vi "Set Cache Params.vi"(8 "error in (no error)":errorcluster, 10 "Cache Params":T1={"Enabled"=FALSE, "Directive"=enum."None (no-store)", "Max Age"=0, "Immutable"=FALSE, "Last Modified"=timestamp(0 s since 1904-01-01), "Expires"=timestamp(0 s since 1904-01-01), "ETag"="", "Weak ETag"=FALSE}, 11 "Response in":refnum<class "Response.lvclass">) -> (0 "error out":errorcluster, 3 "Response out":refnum<class "Response.lvclass">)   [LabVIEW 2020, in "HTTP Utils.lvlib" / "Response.lvclass"]
uses:
  Response.lvclass
  Cache Params.ctl
  Cache Directive.ctl
  HTTP Utils.lvlib
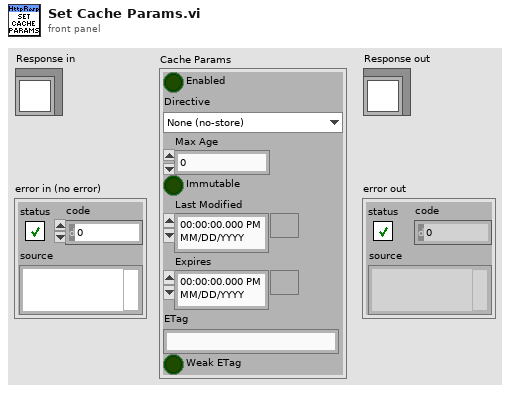
[diagram p1: front panel]
types:
  T1 = typedef "HTTP Utils.lvlib/Cache Params.ctl" = cluster{"Enabled":bool, "Directive":T2, "Max Age":i32, "Immutable":bool, "Last Modified":timestamp, "Expires":timestamp, "ETag":string, "Weak ETag":bool}
  T2 = typedef "HTTP Utils.lvlib/Cache Directive.ctl" = enum16{"Not Specified", "None (no-store)", "Always Validate (no-cache)", "Private Only (private)", "Always Allow (public)"}
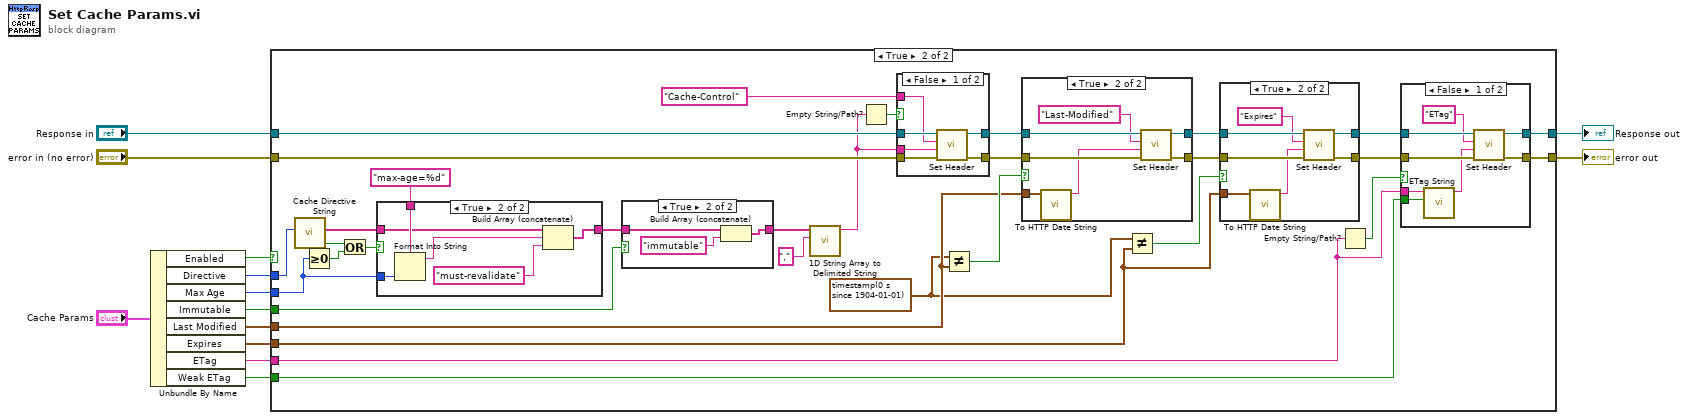
[diagram p0: block diagram]
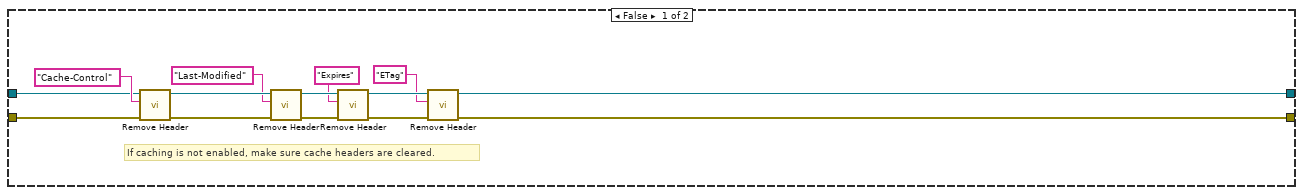
[diagram p2: hidden frame]
diagram:
  n1 = Unbundle By Name("Cache Params") -> ("Enabled"=w12:bool, "Directive"=w11:T2, "Max Age"=w10:i32, "Immutable"=w9:bool, "Last Modified"=w8:timestamp, "Expires"=w7:timestamp, "ETag"=w6:string, "Weak ETag"=w1:bool)
  n2 = case shown="True" w12 {
    tunnel: "error in (no error)" -> [w27 w59]
    tunnel: w11 -> [_ w57]
    tunnel: w10 -> [_ w53]
    tunnel: w9 -> [_ w50]
    tunnel: w8 -> [_ w46]
    tunnel: w7 -> [_ w41]
    tunnel: w6 -> [_ w37]
    tunnel: [w16 w36] -> w5
    tunnel: [w15 w35] -> w4
    tunnel: "Response in" -> [w14 w34]
    tunnel: w1 -> [_ w28]
    frame False {
      # "If caching is not enabled, make sure cache headers are cleared."
      n3 = call "Remove Header.vi"("error in (no error)"=w27, "Header"="Cache-Control", "Response in"=w14) -> ("error out"=w24:errorcluster, "Response out"=w25:refnum<class "Response.lvclass">)  [unwired: 5 in, 2 out]
      n4 = call "Remove Header.vi"("error in (no error)"=w24, "Header"="Last-Modified", "Response in"=w25) -> ("error out"=w21:errorcluster, "Response out"=w22:refnum<class "Response.lvclass">)  [unwired: 5 in, 2 out]
      n5 = call "Remove Header.vi"("error in (no error)"=w21, "Header"="Expires", "Response in"=w22) -> ("error out"=w18:errorcluster, "Response out"=w19:refnum<class "Response.lvclass">)  [unwired: 5 in, 2 out]
      n6 = call "Remove Header.vi"("error in (no error)"=w18, "Header"="ETag", "Response in"=w19) -> ("error out"=w15:errorcluster, "Response out"=w16:refnum<class "Response.lvclass">)  [unwired: 5 in, 2 out]
    }
    frame True {
      w43 = timestamp(0 s since 1904-01-01) ("x")
      n7 = call "Cache Directive String.vi"("Cache Directive"=w57) -> ("Cache-Control Directive"=w56:string[], "no-store?"=w55:bool)  [unwired: 9 in]
      n8 = Greater Or Equal To 0?(x=w53) -> (x >= 0?=w33:bool)
      n9 = Or(x=w55, y=w33) -> (x .or. y?=w54:bool)
      n10 = case shown="True" w54 {
        tunnel: w56 -> [w60 w64]
        tunnel: w53 -> [_ w66]
        tunnel: [w60 w61] -> w51
        tunnel: "max-age=%d" ("string") -> [_ w65]
        frame False {
        }
        frame True {
          n11 = Format Into String(format string=w65, w66) -> (resulting string=w62:string)  [unwired: 2 in, 1 out]
          n12 = Build Array (concatenate)(w64, w62, "must-revalidate" ("string")) -> (w61:string[])
        }
      }
      n13 = case shown="True" w50 {
        tunnel: w51 -> [w103 w106]
        tunnel: [w103 w104] -> w30
        frame False {
        }
        frame True {
          n14 = Build Array (concatenate)(w106, "immutable" ("string")) -> (w104:string[])
        }
      }
      n15 = call <vilib>:"1D String Array to Delimited String.vi"("delimiter"=",", "string array"=w30) -> ("delimited string"=w29:string)  [unwired: 9 in]
      n16 = Empty String/Path?(string/path=w29) -> (empty?=w32:bool)
      n17 = case shown="False" w32 {
        tunnel: w59 -> [w72 w73]
        tunnel: "Cache-Control" ("Header") -> [w67 _]
        tunnel: w29 -> [w71 _]
        tunnel: [w70 w74] -> w48
        tunnel: [w69 w73] -> w47
        tunnel: w34 -> [w68 w74]
        frame False {
          n18 = call "Set Header.vi"("error in (no error)"=w72, "Value"=w71, "Header"=w67, "Response in"=w68) -> ("error out"=w69:errorcluster, "Response out"=w70:refnum<class "Response.lvclass">)  [unwired: 5 in, 1 out]
        }
        frame True {
        }
      }
      n19 = Not Equal?(x=w43, y=w46) -> (x != y?=w49:bool)
      n20 = case shown="True" w49 {
        tunnel: w48 -> [w94 w102]
        tunnel: w47 -> [w95 w101]
        tunnel: w46 -> [_ w99]
        tunnel: [w94 w97] -> w44
        tunnel: [w95 w96] -> w45
        frame False {
        }
        frame True {
          n21 = call "To HTTP Date String.vi"("Time Stamp"=w99) -> ("HTTP Date"=w98:string)  [unwired: 10 in]
          n22 = call "Set Header.vi"("error in (no error)"=w101, "Value"=w98, "Header"="Last-Modified", "Response in"=w102) -> ("error out"=w96:errorcluster, "Response out"=w97:refnum<class "Response.lvclass">)  [unwired: 5 in, 1 out]
        }
      }
      n23 = Not Equal?(x=w43, y=w41) -> (x != y?=w42:bool)
      n24 = case shown="True" w42 {
        tunnel: w45 -> [w85 w91]
        tunnel: w44 -> [w86 w92]
        tunnel: w41 -> [_ w93]
        tunnel: [w86 w88] -> w40
        tunnel: [w85 w87] -> w39
        frame False {
        }
        frame True {
          n25 = call "To HTTP Date String.vi"("Time Stamp"=w93) -> ("HTTP Date"=w90:string)  [unwired: 10 in]
          n26 = call "Set Header.vi"("error in (no error)"=w91, "Value"=w90, "Header"="Expires", "Response in"=w92) -> ("error out"=w87:errorcluster, "Response out"=w88:refnum<class "Response.lvclass">)  [unwired: 5 in, 1 out]
        }
      }
      n27 = Empty String/Path?(string/path=w37) -> (empty?=w38:bool)
      n28 = case shown="False" w38 {
        tunnel: w40 -> [w82 w84]
        tunnel: w39 -> [w81 w83]
        tunnel: w37 -> [w77 _]
        tunnel: [w79 w84] -> w36
        tunnel: [w78 w83] -> w35
        tunnel: w28 -> [w76 _]
        frame False {
          n29 = call "ETag String.vi"("Weak"=w76, "ETag"=w77) -> ("ETag Value"=w75:string)  [unwired: 9 in]
          n30 = call "Set Header.vi"("error in (no error)"=w81, "Value"=w75, "Header"="ETag", "Response in"=w82) -> ("error out"=w78:errorcluster, "Response out"=w79:refnum<class "Response.lvclass">)  [unwired: 5 in, 1 out]
        }
        frame True {
        }
      }
    }
  }
  "error out" <- w4
  "Response out" <- w5
